vi "Compute Weight Array v2.vi"(8 "Error In":errorcluster, 9 "Weighted Fit":T1, 10 "Control Data Array":dbl[](array[numeric]), 11 "Data Array":dbl[](array[numeric])) -> (0 "Error Out":errorcluster, 3 "Weight Array":dbl[](array[numeric]))   [LabVIEW 2021, in "Fits.lvlib"]
doc: "If provided, the control array should have the same dimension as the data array and be in [0, 1]"
uses:
  Fits.lvlib
  IRF(X)PSED/Fit Weights Type v2.ctl
  <userlib>/_OpenG.lib/array/array.llb/Filter 1D Array with Scalar (DBL)__ogtk.vi
  Arrays/Arrays.lvlib
  <userlib>/_OpenG.lib/array/array.llb/openg_array.lvlib
panel:
  # "<--------- between 0 and 1"
  # "see the License on the block diagram (Ctrl+E or Window:Show Block Diagram)"
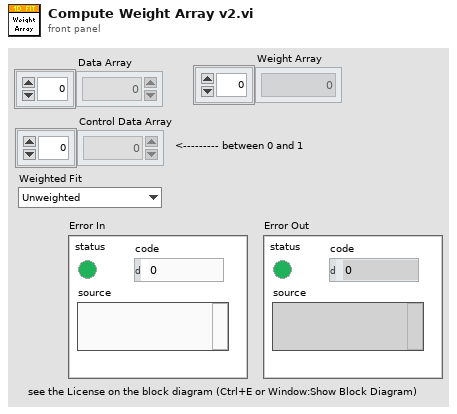
[diagram p1: front panel]
types:
  T1 = typedef "Fits.lvlib/Fit Weights Type v2.ctl" = enum16{"Unweighted", "1/Variance (Neyman)", "1/Variance (Pearson)", "Best of All"}
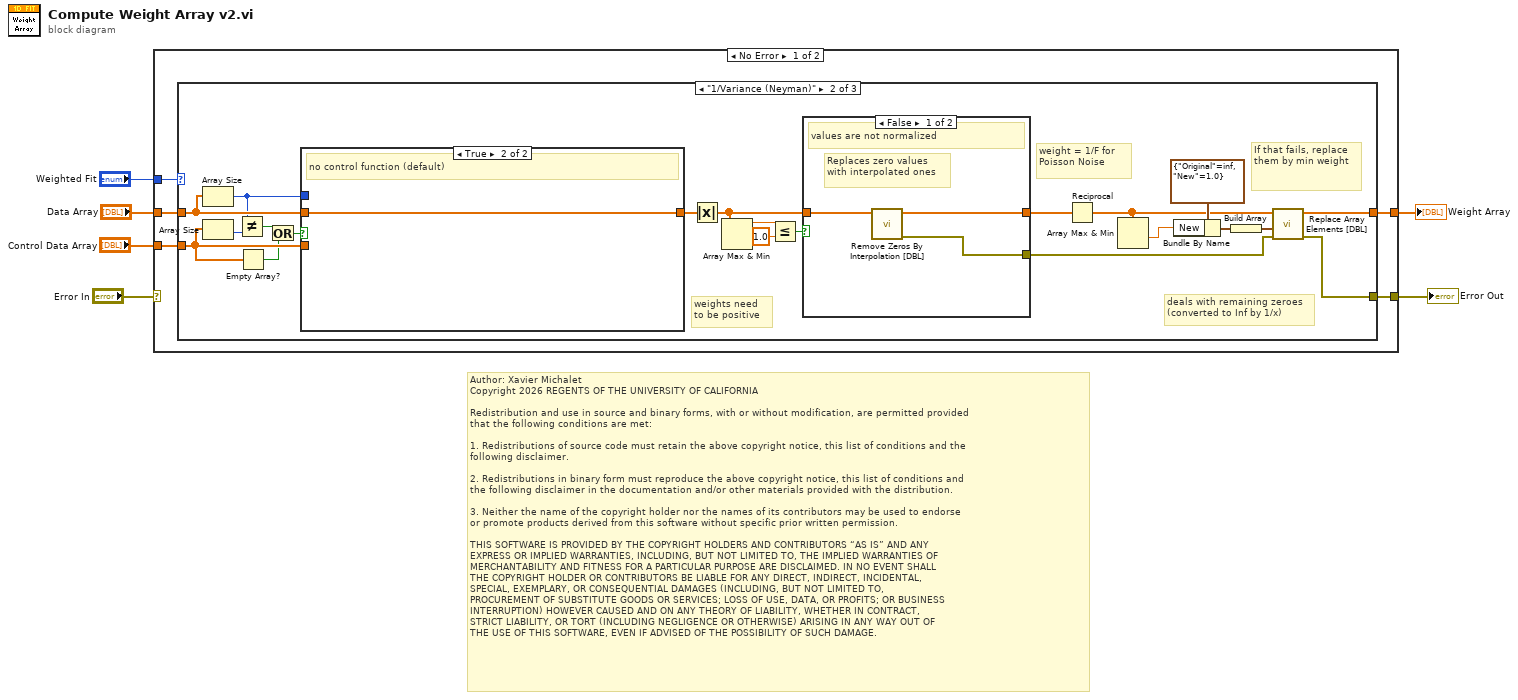
[diagram p0: block diagram]
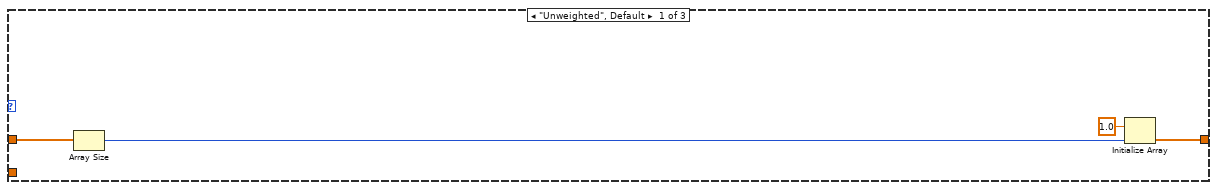
[diagram p2: hidden frame]
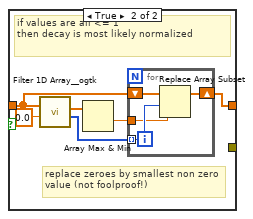
[diagram p3: hidden frame]
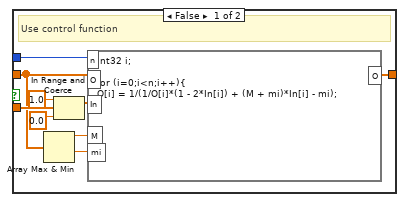
[diagram p4: hidden frame]
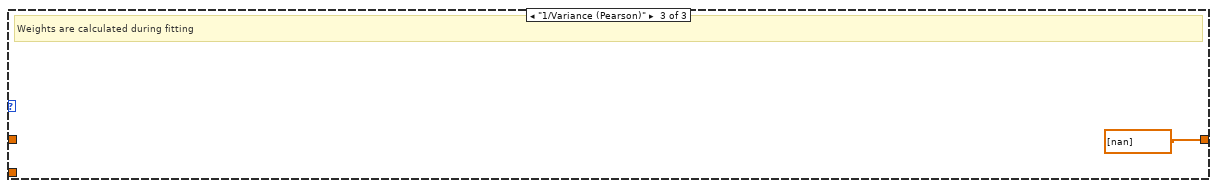
[diagram p5: hidden frame]
diagram:
  # "Author: Xavier Michalet\nCopyright 2026 REGENTS OF THE UNIVERSITY OF CALIFORNIA\n\nRedistribution and use in source and binary forms, with or without modification, are permitted provided\nthat the following conditions are met:\n\n1. Redistributions of source code must retain the above copyright notice, this list of conditions and the\nfollowing disclaimer.\n\n2. Redistributions in binary form must reproduce the above copyright notice, this list of conditions and\nthe following disclaimer in the documentation and/or other materials provided with the distribution.\n\n3. Neither the name of the copyright holder nor the names of its contributors may be used to endorse \nor promote products derived from this software without specific prior written permission.\n\nTHIS SOFTWARE IS PROVIDED BY THE COPYRIGHT HOLDERS AND CONTRIBUTORS “AS IS” AND ANY \nEXPRESS OR IMPLIED WARRANTIES, INCLUDING, BUT NOT LIMITED TO, THE IMPLIED WARRANTIES OF\nMERCHANTABILITY AND FITNESS FOR A PARTICULAR PURPOSE ARE DISCLAIMED. IN NO EVENT SHALL\nTHE COPYRIGHT HOLDER OR CONTRIBUTORS BE LIABLE FOR ANY DIRECT, INDIRECT, INCIDENTAL, \nSPECIAL, EXEMPLARY, OR CONSEQUENTIAL DAMAGES (INCLUDING, BUT NOT LIMITED TO, \nPROCUREMENT OF SUBSTITUTE GOODS OR SERVICES; LOSS OF USE, DATA, OR PROFITS; OR BUSINESS\nINTERRUPTION) HOWEVER CAUSED AND ON ANY THEORY OF LIABILITY, WHETHER IN CONTRACT, \nSTRICT LIABILITY, OR TORT (INCLUDING NEGLIGENCE OR OTHERWISE) ARISING IN ANY WAY OUT OF\nTHE USE OF THIS SOFTWARE, EVEN IF ADVISED OF THE POSSIBILITY OF SUCH DAMAGE."
  n1 = case shown="No Error" "Error In" {
    selector: "Error In" -> [_ w60]
    tunnel: [w11 _] -> w6
    tunnel: "Data Array" -> [w9 _]
    tunnel: "Weighted Fit" -> [w10 _]
    tunnel: "Control Data Array" -> [w8 _]
    tunnel: [w7 w60] -> w1
    frame No Error {
      n2 = case shown="\"1/Variance (Neyman)\"" w10 {
        tunnel: [w15 w35 dbl[] [nan] ("Array with Replacements")] -> w11
        tunnel: w9 -> [w13 w34 _]
        tunnel: w8 -> [_ w33 _]
        tunnel: [_ w21 _] -> w7
        frame "Unweighted", Default {
          n3 = Array Size(array=w13) -> (size(s)=w12:i32)
          n4 = Initialize Array(1.0 ("element"), w12) -> (w15:dbl[])
        }
        frame "1/Variance (Neyman)" {
          w27 = cluster{"Original":dbl, "New":dbl} {"Original"=inf, "New"=1.0} ("Array of Replacement Pairs")
          # "deals with remaining zeroes\n(converted to Inf by 1/x)"
          # "weight = 1/F for Poisson Noise"
          # "weights need to be positive"
          # "If that fails, replace them by min weight"
          n5 = Array Size(array=w34) -> (size(s)=w28:i32)
          n6 = Array Size(array=w33) -> (size(s)=w32:i32)
          n7 = Not Equal?(x=w28, y=w32) -> (x != y?=w31:bool)
          n8 = Empty Array?(array=w33) -> (empty?=w30:bool)
          n9 = Or(x=w31, y=w30) -> (x .or. y?=w29:bool)
          n10 = case shown="True" w29 {
            tunnel: w34 -> [w51 w58]
            tunnel: [w52 w58] -> w20
            tunnel: w33 -> [w57 _]
            tunnel: w28 -> [w53 _]
            frame False {
              # "Use control function"
              n11 = Array Max & Min(array=w51) -> (max value=w50:dbl, min value=w49:dbl)  [unwired: 2 out]
              n12 = In Range and Coerce(upper limit=1.0, x=w57, lower limit=0.0 ("upper limit")) -> (coerced(x)=w54:dbl[])  [unwired: 1 out]
              n13 = formula code="int32 i;\n\nfor (i=0;i<n;i++){\nO[i] = 1/(1/O[i]*(1 - 2*In[i]) + (M + mi)*In[i] - mi);\n}"("O"=w51, "In"=w54, "n"=w53, "M"=w50, "mi"=w49) -> ("O"=w52:dbl[])
            }
            frame True {
              # "no control function (default)"
            }
          }
          n14 = Absolute Value(x=w20) -> (abs(x)=w19:dbl[])
          n15 = Array Max & Min(array=w19) -> (max value=w18:dbl)  [unwired: 3 out]
          n16 = Less Or Equal?(x=w18, y=1.0) -> (x <= y?=w16:bool)
          n17 = case shown="False" w16 {
            tunnel: [w38 w39] -> w25
            tunnel: [w37 _] -> w22
            tunnel: w19 -> [w36 w42]
            frame False {
              # "Replaces zero values with interpolated ones"
              # "values are not normalized"
              n18 = call "Remove Zeros By Interpolation [DBL].vi"("Array in"=w36) -> ("Error Out"=w37:errorcluster, "Array out"=w38:dbl[])  [unwired: 9 in]
            }
            frame True {
              # "replace zeroes by smallest non zero value (not foolproof!)"
              # "if values are all <= 1\nthen decay is most likely normalized"
              n19 = call-poly <userlib>:"Filter 1D Array__ogtk.vi"("items to filter"=0.0 ("Numeric Control"), "array"=w42) -> ("filtered item indices"=w40:i32[], "filtered array"=w43:dbl[])  [unwired: 4 in]
              n20 = Array Max & Min(array=w43) -> (min value=w41:dbl)  [unwired: 3 out]
              n21 = for {
                shift-right: [w47] -> w39
                shift-left: w42 -> [w48]
                tunnel: w41 -> [w45]
                tunnel: w40 -> [w46] mode=indexing
                n22 = Replace Array Subset(array=w48, new element=w45, index=w46) -> (w47:dbl[])
              }
            }
          }
          n23 = Reciprocal(x=w25) -> (1/x=w24:dbl[])
          n24 = Array Max & Min(array=w24) -> (min value=w23:dbl)  [unwired: 3 out]
          n25 = Bundle By Name(cluster=w27, "New"=w23) -> ()  [unwired: 1 out]
          n26 = Build Array(w27) -> (w26:cluster{"Original":dbl, "New":dbl}[])
          n27 = call "Replace Array Elements [DBL].vi"("Error In"=w22, "Array of Replacement Pairs"=w26, "Array"=w24) -> ("Error Out"=w21:errorcluster, "Array with Replacements"=w35:dbl[])  [unwired: 7 in]
        }
        frame "1/Variance (Pearson)" {
          # "Weights are calculated during fitting"
        }
      }
    }
    frame Error {
    }
  }
  "Weight Array" <- w6
  "Error Out" <- w1
